vi "Midterm Spectral AnalyzerV2.vi"() -> ()   [LabVIEW 2022 SP3]
uses:
  <vilib>/express/express analysis/Spectral/Block/exnSpectralBlock spectral measurements power poly.vi
  <vilib>/express/express analysis/Spectral/Block/exnSpectralBlock spectral measurements power DDT.vi
  <vilib>/express/express analysis/Spectral/XNode/ExpressSpectralMeasurementsBlockNode.xnode
  <vilib>/Analysis/NI_AAL_SigProc.lvlib
panel:
  in  "Tab Control":enum32{"Page 1", "Page 2"}(tab)
  in  "?":bool
  in  "?":bool
  in  "?":bool
  in  "?":bool
  in  "Sound File Path":path
  out "Spectral Information (Power Spectrum)":dynamicdata(graph)
  out "Raw Waveform":dynamicdata(graph)
  out "Fundamental":dbl
  out "Loudest":dbl
  out "Max Indx":i32
  out "max value":dbl
  in  "stop":bool
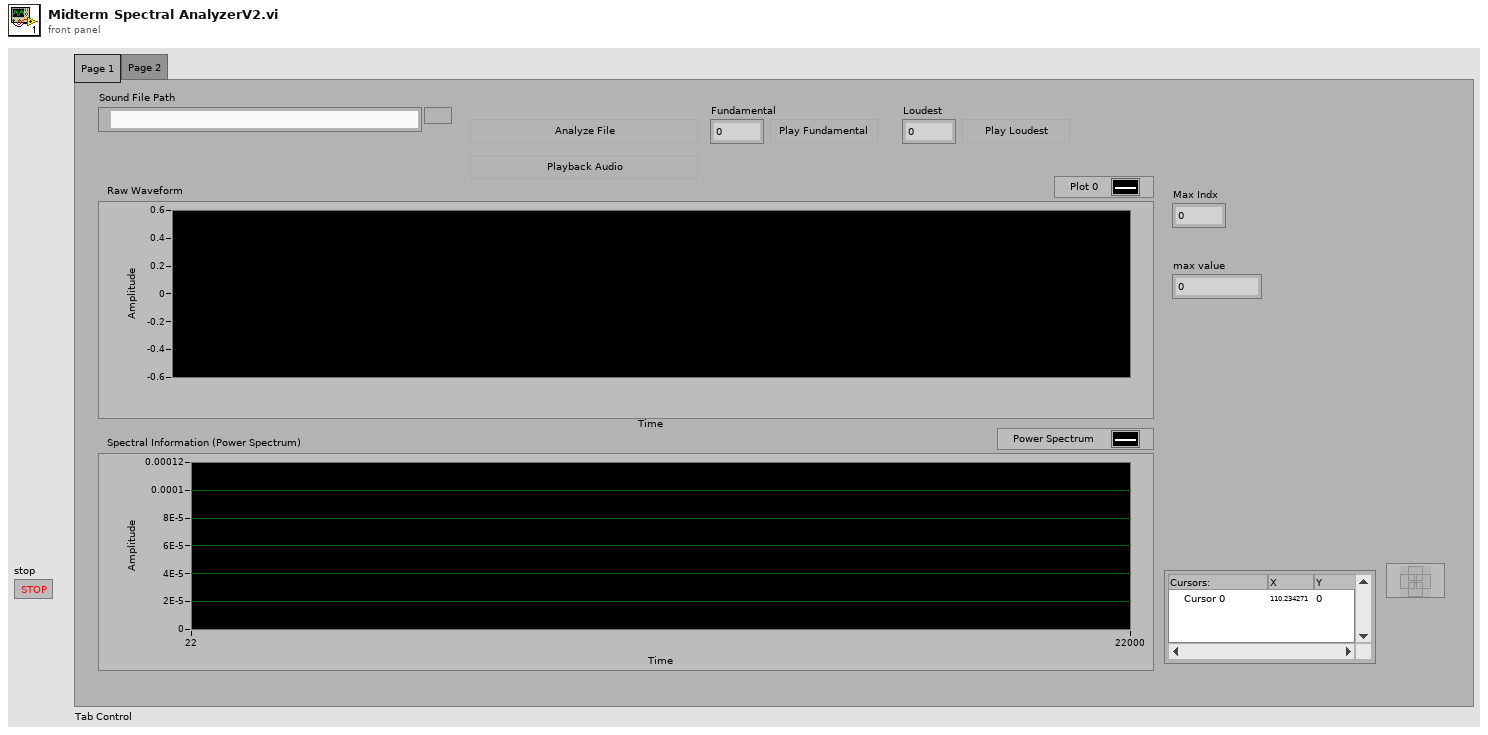
[diagram p1: front panel]
types:
  T1 = cluster{"averaging mode":u16, "weighting mode":u16, "number of averages":u32}
  T2 = cluster{"dB On (F)":bool, "unwrap phase (F)":bool, "convert to degree (F)":bool}
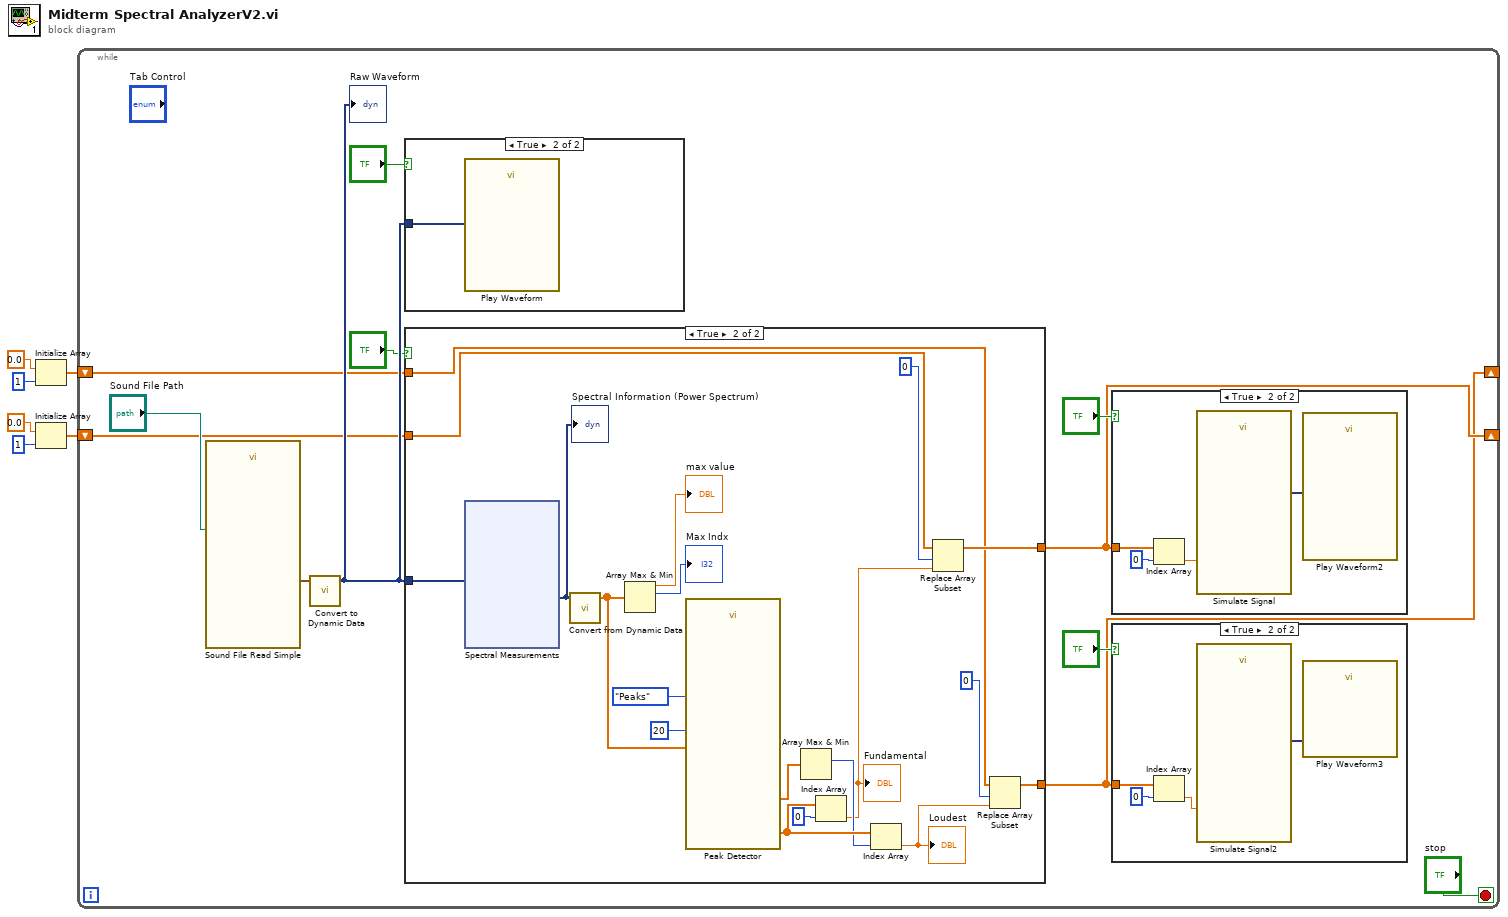
[diagram p0: block diagram]
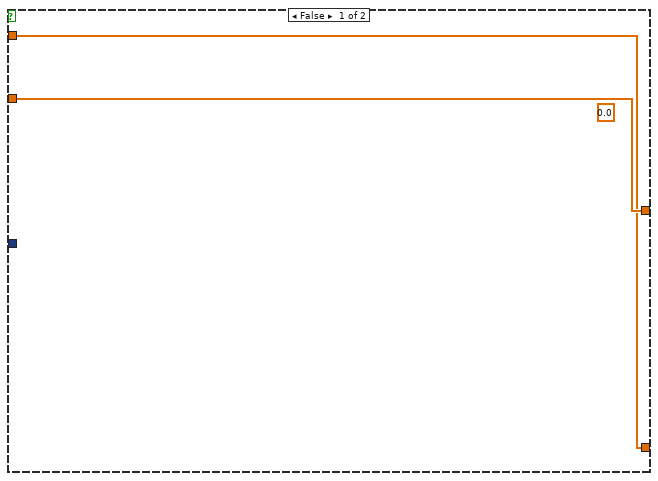
[diagram p4: hidden frame]
diagram:
  n1 = Initialize Array(0.0 ("element"), 1 ("dimension size")) -> (w3:dbl[])
  n2 = Initialize Array(0.0 ("element"), 1 ("dimension size")) -> (w4:dbl[])
  n3 = while {
    shift-right: [w8] -> _
    shift-left: w4 -> [w10]
    shift-right: [w7] -> _
    shift-left: w3 -> [w9]
    stop <- "stop" stop-if-true
    n4 = call <vilib>:"Sound File Read Simple.vi"("path"="Sound File Path") -> ("data"=w15:waveform(dbl)[])  [unwired: 7 in, 3 out]
    n5 = call "Convert to Dynamic Data"("Array of Waveforms"=w15) -> ("Dynamic Data Type"=w17:dynamicdata)  [unwired: 3 in]
    "Raw Waveform" <- w17
    n6 = case shown="True" "?" {
      tunnel: w17 -> [_ w57]
      frame False {
      }
      frame True {
        n7 = call "Play Waveform"("Data"=w57) -> ()  [unwired: 18 in, 1 out]
      }
    }
    n8 = case shown="True" "?" {
      tunnel: w17 -> [_ w47]
      tunnel: [w27 w29] -> w7
      tunnel: w10 -> [w28 w36]
      tunnel: [w28 w33] -> w8
      tunnel: w9 -> [w27 w31]
      frame False {
        (unwired) 0.0
      }
      frame True {
        n9 = xnode "Spectral Measurements"("Signals"=w47) -> ("Power Spectrum"=w46:dynamicdata)  [unwired: 1 in, 1 out]
        "Spectral Information (Power Spectrum)" <- w46
        n10 = call "Convert from Dynamic Data"("Dynamic Data Type"=w46) -> ("Array"=w39:dbl[])  [unwired: 3 in]
        n11 = Array Max & Min(array=w39) -> (max value=→"max value":dbl, max index (indices)=→"Max Indx":i32)  [unwired: 2 out]
        n12 = call <vilib>:"Peak Detector.vi"("peaks/valleys"=enum32{"Peaks", "Valleys"}."Peaks", "width"=20, "X"=w39) -> ("Amplitudes"=w42:dbl[], "Locations"=w44:dbl[])  [unwired: 4 in, 3 out]
        n13 = Array Max & Min(array=w42) -> (max index (indices)=w41:i32)  [unwired: 3 out]
        n14 = Index Array(array=w44, index=0) -> (element=w35:dbl)
        "Fundamental" <- w35
        n15 = Index Array(array=w44, index=w41) -> (element=w30:dbl)
        "Loudest" <- w30
        n16 = Replace Array Subset(array=w36, new element=w35, index=0) -> (w33:dbl[])
        n17 = Replace Array Subset(array=w31, new element=w30, index=0) -> (w29:dbl[])
      }
    }
    n18 = case shown="True" "?" {
      tunnel: w8 -> [_ w24]
      frame False {
      }
      frame True {
        n19 = Index Array(array=w24, index=0) -> (element=w23:dbl)
        n20 = call "Simulate Signal"("Frequency"=w23) -> ("Sine"=w26:dynamicdata)  [unwired: 13 in, 1 out]
        n21 = call "Play Waveform2"("Data"=w26) -> ()  [unwired: 18 in, 1 out]
      }
    }
    n22 = case shown="True" "?" {
      tunnel: w7 -> [_ w19]
      frame False {
      }
      frame True {
        n23 = Index Array(array=w19, index=0) -> (element=w20:dbl)
        n24 = call "Simulate Signal2"("Frequency"=w20) -> ("Sine"=w22:dynamicdata)  [unwired: 13 in, 1 out]
        n25 = call "Play Waveform3"("Data"=w22) -> ()  [unwired: 18 in, 1 out]
      }
    }
  }
